vi "practica2_ejercicio3.vi"(0 "INDICE":dbl, 2 "TAM_SUB":dbl, 3 "TAMAÑO":dbl) -> (1 "RAIZ CUADRADA":dbl[](array[numeric]), 4 "SUBCONJUNTO":dbl[](array[numeric]), 5 "ORDENADOS":dbl[](array[numeric]), 6 "DECIMALES":dbl[](array[numeric]), 7 "ENTEROS":dbl[](array[numeric]))   [LabVIEW 2011]
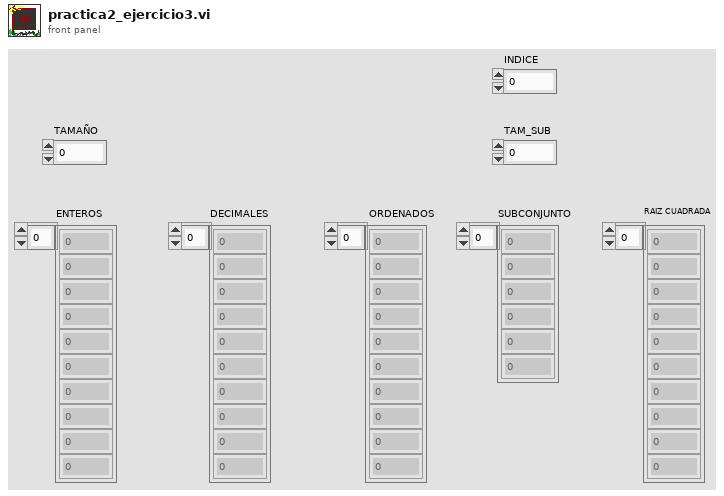
[diagram p1: front panel]
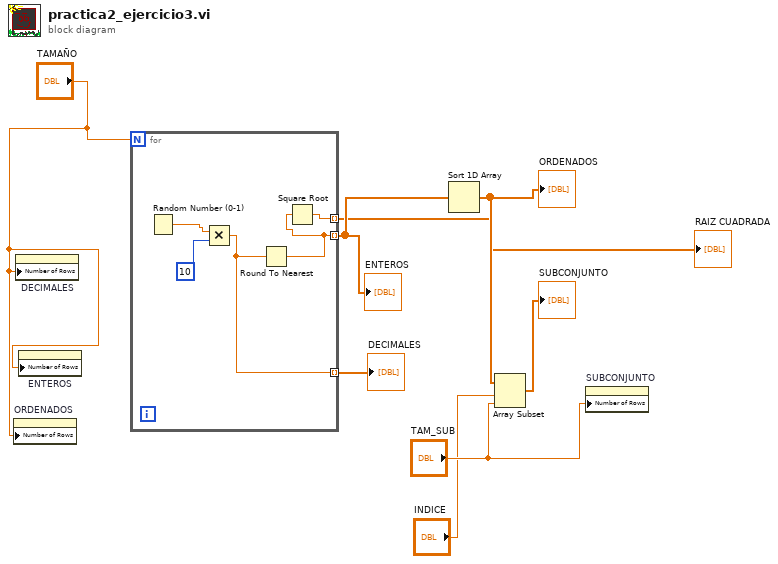
[diagram p0: block diagram]
diagram:
  n1 = property on="ORDENADOS" class="Arr (strict)"("Number of Rows"="TAMAÑO") -> ()  [unwired: 2 in, 2 out]
  n2 = property on="DECIMALES" class="Arr (strict)"("Number of Rows"="TAMAÑO") -> ()  [unwired: 2 in, 2 out]
  n3 = property on="ENTEROS" class="Arr (strict)"("Number of Rows"="TAMAÑO") -> ()  [unwired: 2 in, 2 out]
  n4 = for {
    N: "TAMAÑO" -> [_]
    tunnel: [w10] -> w7 mode=indexing
    tunnel: [w11] -> w8 mode=indexing
    tunnel: [w9] -> w3 mode=indexing
    n5 = Random Number (0-1)() -> (number: 0 to 1=w13:dbl)
    n6 = Multiply(x=w13, y=10) -> (x*y=w11:dbl)
    n7 = Round To Nearest(number=w11) -> (nearest integer value=w10:dbl)
    n8 = Square Root(x=w10) -> (sqrt(x)=w9:dbl)
  }
  "DECIMALES" <- w8
  "ENTEROS" <- w7
  "RAIZ CUADRADA" <- w3
  n9 = Sort 1D Array(array=w7) -> (sorted array=w6:dbl[])
  "ORDENADOS" <- w6
  n10 = Array Subset(array=w6, index="INDICE", length="TAM_SUB") -> (→"SUBCONJUNTO":dbl[])
  n11 = property on="SUBCONJUNTO" class="Arr (strict)"("Number of Rows"="TAM_SUB") -> ()  [unwired: 2 in, 2 out]
